vi "Write initialized.vi"(8 "error in (no error)":errorcluster, 10 "initialized":bool, 11 "Socket.Base in":refnum<class "Socket.Base.lvclass">) -> (0 "error out":errorcluster, 3 "Socket.Base out":refnum<class "Socket.Base.lvclass">)   [LabVIEW 2014, in "Socket.lvlib" / "Socket.Base.lvclass"]
uses:
  Socket.Base.lvclass
  Socket.Base.lvclass/Socket.Base.ctl
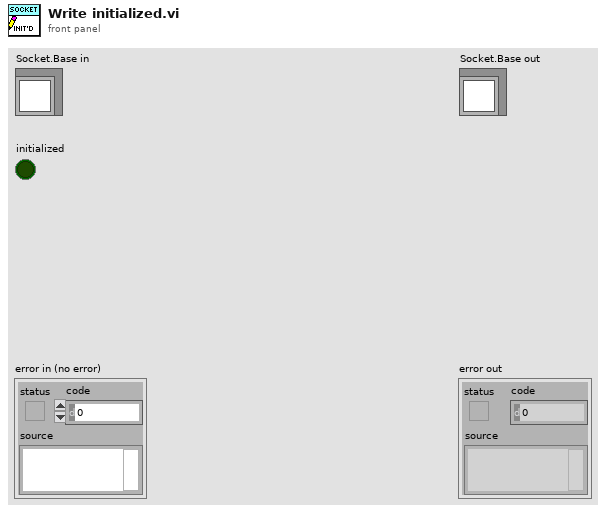
[diagram p1: front panel]
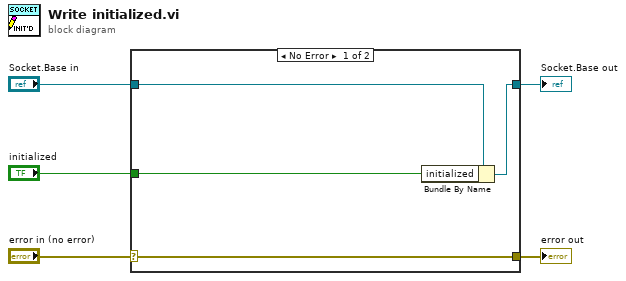
[diagram p0: block diagram]
diagram:
  n1 = case shown="No Error" "error in (no error)" {
    selector: "error in (no error)" -> [w9 w10]
    tunnel: [w9 w10] -> w4
    tunnel: [w7 w11] -> w2
    tunnel: "Socket.Base in" -> [w8 w11]
    tunnel: "initialized" -> [w6 _]
    frame No Error {
      n2 = Bundle By Name(cluster=w8, "initialized"=w6) -> (w7:refnum<class "Socket.Base.lvclass">)
    }
    frame Error {
    }
  }
  "error out" <- w4
  "Socket.Base out" <- w2
